vi "wait_globals.vi"() -> ()   [LabVIEW 2011]
panel:
  out "Initial time":timestamp
  in  "Wait time remaining (s)":dbl
  out "Total wait time (m:s)":string
  in  "Total wait time (s)":dbl
  in  "Done":bool
  out "Wait time remaining (m:s)":string
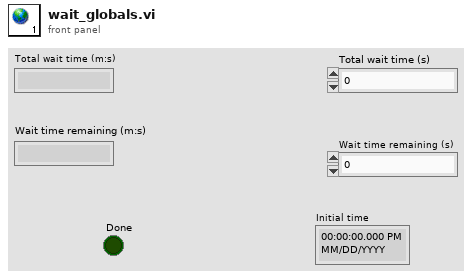
[diagram p1: front panel]
diagram:
